vi "Push the Rock.vi"(0 "Move #Units per Push":i32, 1 "Rock Position in Chamber in":i32=3, 2 "Chamber":u32[][](array[colorbox]), 4 "Rock in":u32[][](array[colorbox]), 5 "Push Direction":u8, 6 "Consider Wall Boundary ? (T)":bool=TRUE) -> (7 "Rock out":u32[][](array[colorbox]))   [LabVIEW 2020, in "AoC 2022.lvlib"]
uses:
  AoC 2022.lvlib
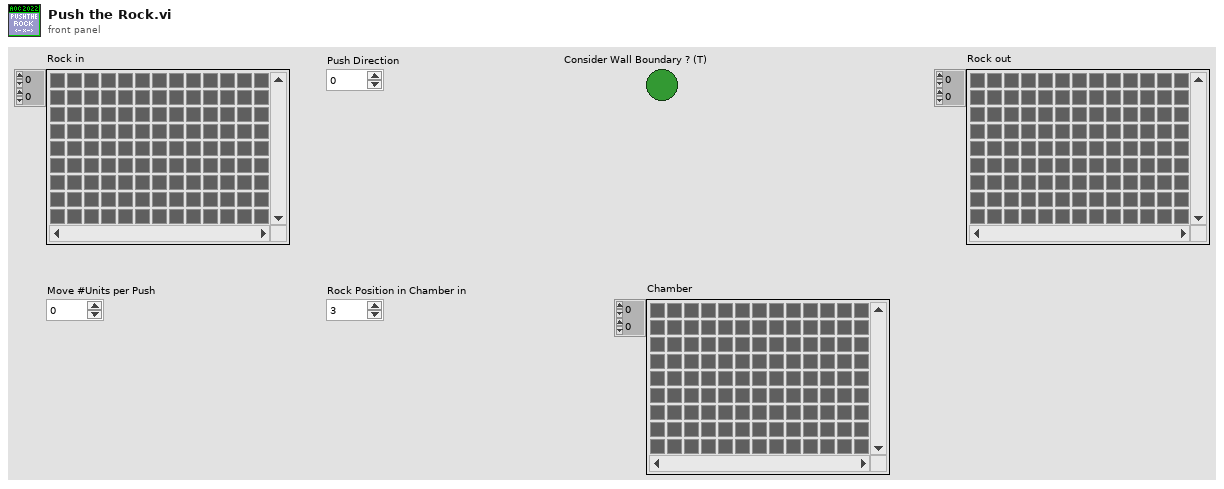
[diagram p1: front panel]
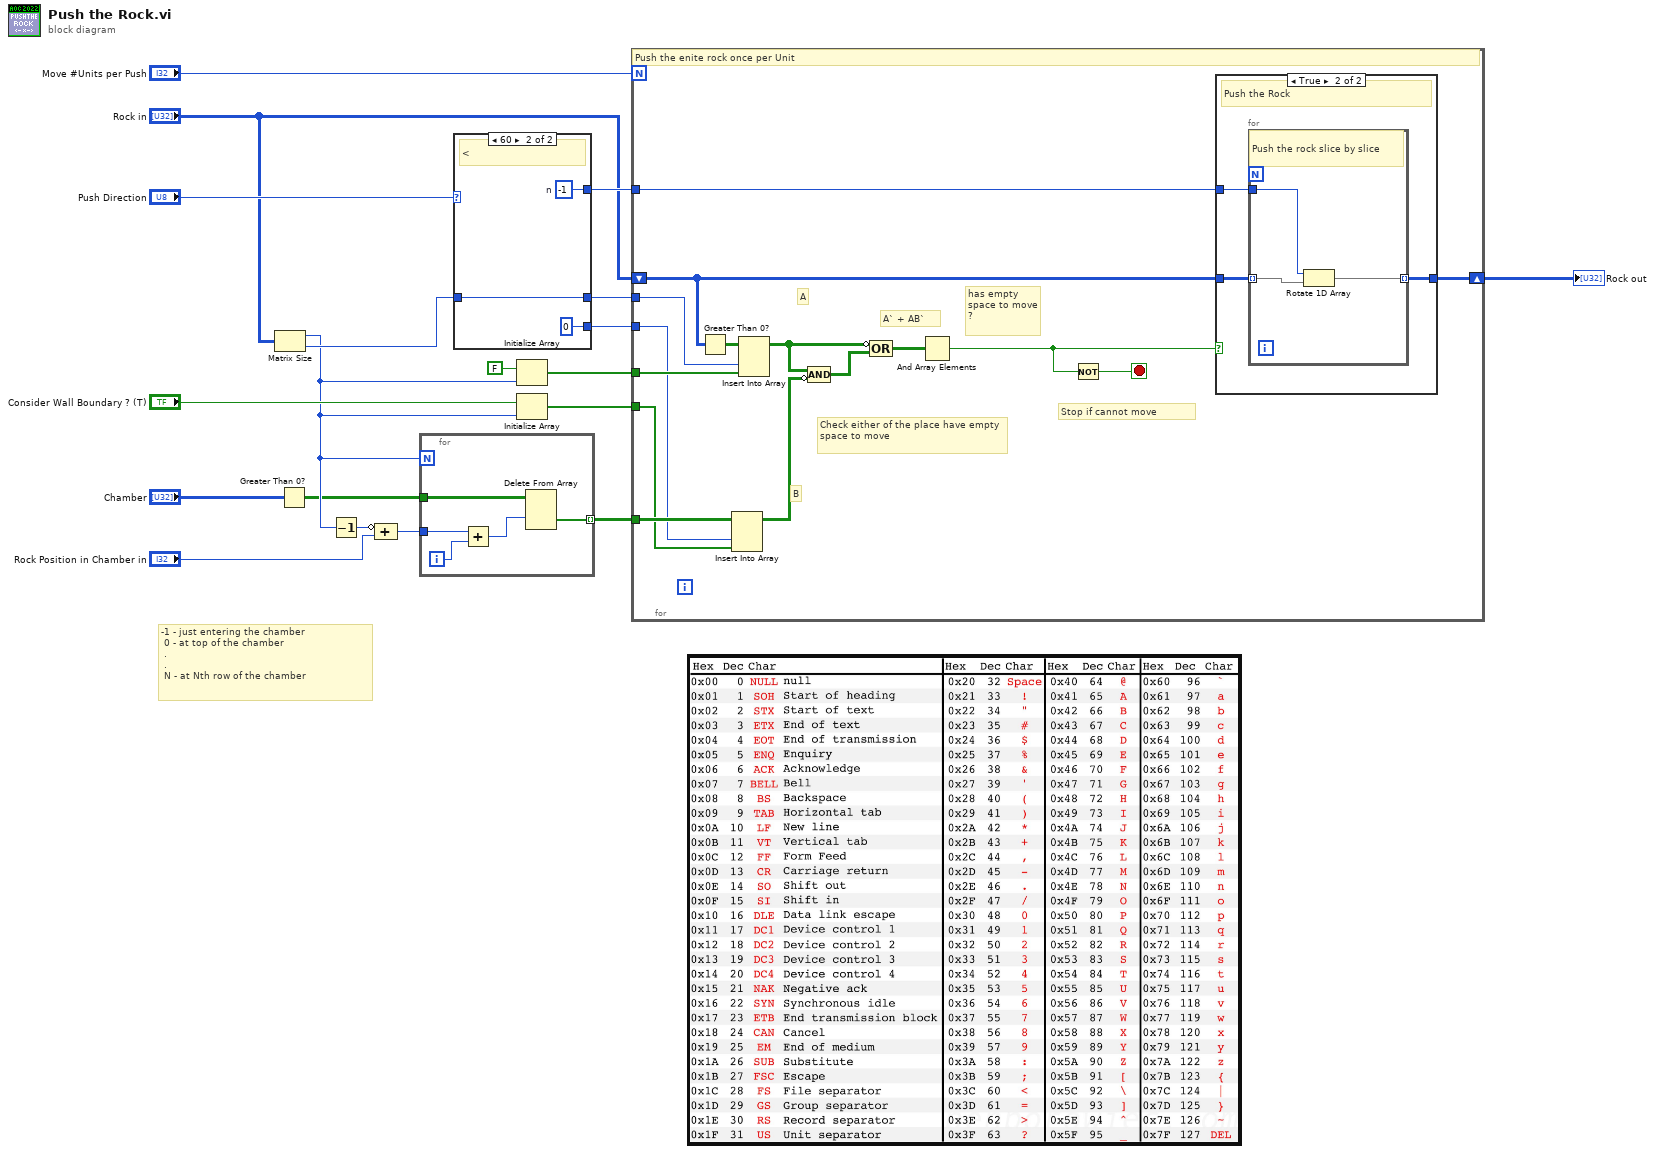
[diagram p0: block diagram]
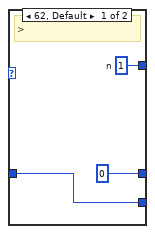
[diagram p2: hidden frame]
diagram:
  # "-1 - just entering the chamber\n 0 - at top of the chamber\n .\n .\n N - at Nth row of the chamber"
  n1 = Matrix Size(0:"Rock in") -> (1:w4:i32, 2:w7:i32)
  n2 = Greater Than 0?(x="Chamber") -> (x > 0?=w1:bool[][])
  n3 = Decrement(x=w4) -> (x-1=w14:i32)
  n4 = Compound Arithmetic op=ADD(invert w14, "Rock Position in Chamber in") -> (w3:i32)
  n5 = for {
    N: w4 -> [_]
    tunnel: [w24] -> w13 mode=indexing
    tunnel: w1 -> [w23]
    tunnel: w3 -> [w21]
    i -> [w22]
    n6 = Add(x=w21, y=w22) -> (x+y=w20:i32)
    n7 = Delete From Array(array=w23, index (row)=w20) -> (deleted portion=w24:bool[])  [unwired: 2 in, 1 out]
  }
  n8 = case shown="60" "Push Direction" {
    tunnel: [w27 w30] -> w19
    tunnel: [0 w29] -> w8
    tunnel: w7 -> [w25 w29]
    tunnel: [w25 0] -> w6
    frame 62, Default {
      w27 = 1  # n
      # ">"
    }
    frame 60 {
      w30 = -1  # n
      # "<"
    }
  }
  n9 = Initialize Array(FALSE, w4) -> (w11:bool[])
  n10 = Initialize Array("Consider Wall Boundary ? (T)", w4) -> (w9:bool[])
  n11 = for {
    N: "Move #Units per Push" -> [_]
    shift-right: [w42] -> w17
    shift-left: "Rock in" -> [w43]
    tunnel: w13 -> [w45]
    tunnel: w19 -> [w41]
    tunnel: w11 -> [w35]
    tunnel: w9 -> [w34]
    tunnel: w8 -> [w33]
    tunnel: w6 -> [w32]
    stop <- w40 stop-if-true
    # "Stop if cannot move"
    # "A` + AB`"
    # "B"
    # "A"
    # "has empty space to move ?"
    # "Check either of the place have empty space to move"
    # "Push the enite rock once per Unit"
    n12 = Greater Than 0?(x=w43) -> (x > 0?=w31:bool[][])
    n13 = Insert Into Array(array=w45, index (col)=w32, new element=w34) -> (w38:bool[][])  [unwired: 1 in]
    n14 = Insert Into Array(array=w31, index (col)=w33, new element=w35) -> (w36:bool[][])  [unwired: 1 in]
    n15 = Compound Arithmetic op=AND(w36, invert w38) -> (w39:bool[][])
    n16 = Compound Arithmetic op=OR(invert w36, w39) -> (w44:bool[][])
    n17 = And Array Elements(Boolean array=w44) -> (logical AND=w37:bool)
    n18 = Not(x=w37) -> (.not. x?=w40:bool)
    n19 = case shown="True" w37 {
      tunnel: w43 -> [w46 w49]
      tunnel: [w46 w48] -> w42
      tunnel: w41 -> [_ w47]
      frame False {
        # "Hit some boundary"
      }
      frame True {
        # "Push the Rock"
        n20 = for {
          tunnel: w49 -> [w52] mode=indexing
          tunnel: [w51] -> w48 mode=indexing
          tunnel: w47 -> [w50]
          # "Push the rock slice by slice"
          n21 = Rotate 1D Array(1:w52, 2:w50) -> (0:w51:u32[])
        }
      }
    }
  }
  "Rock out" <- w17
